vi "rango_dB.vi"(10 "rangosDB in":string[][](array[string])=[["50", "140"], ["40", "130"]], 11 "referencia[dB]":dbl format="%#_13g") -> (0 "tablaRef (Num)":dbl[](array[numeric]), 2 "Referencia[dB]":string[](array[string]), 3 "rango[dB]":string[](array[string]))   [LabVIEW 2019, in "Prueba07.lvclass"]
uses:
  Prueba07.lvclass
panel:
  out "ref_BD":string[](array[string])
  out "ref_NivMax":string[](array[string])
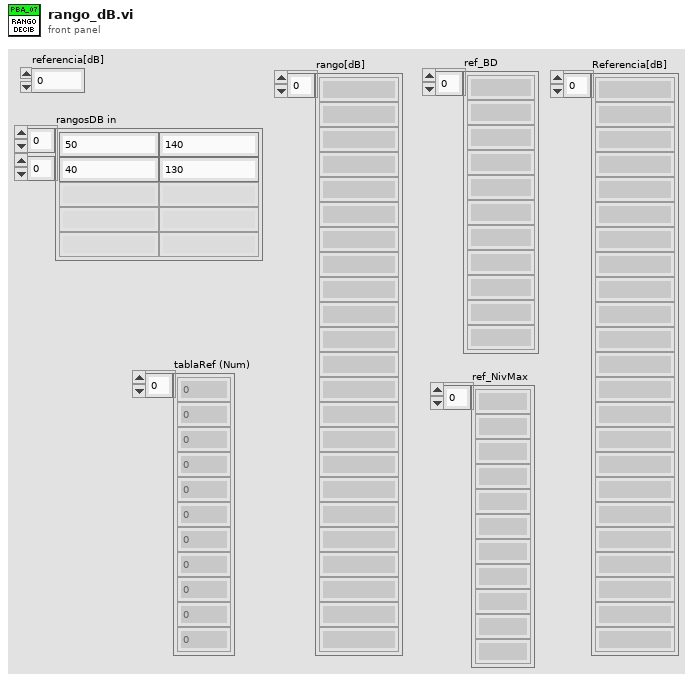
[diagram p1: front panel]
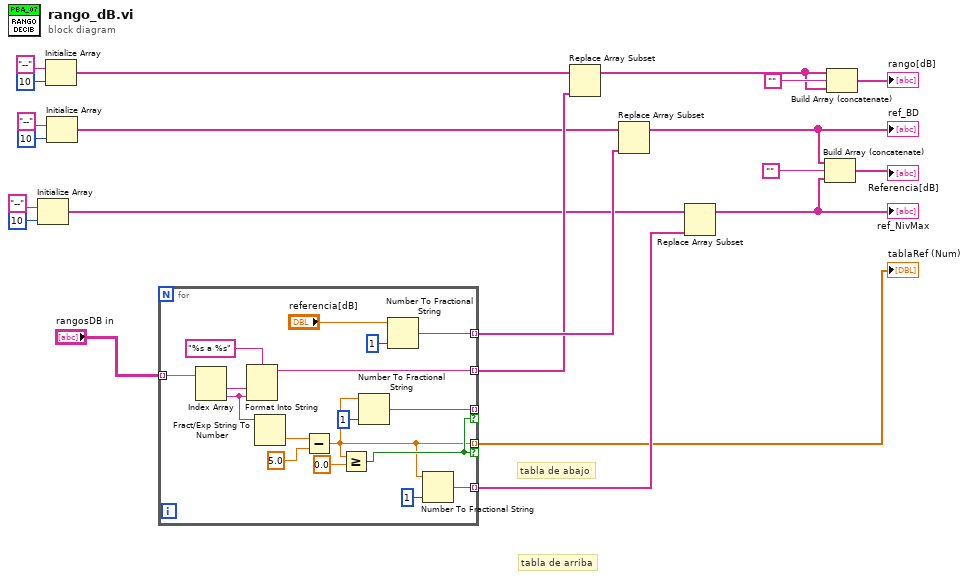
[diagram p0: block diagram]
diagram:
  # "tabla de abajo"
  # "tabla de arriba"
  n1 = Initialize Array("--" ("format string"), 10 ("dimension size")) -> (w6:string[])
  n2 = Initialize Array("--" ("format string"), 10 ("dimension size")) -> (w4:string[])
  n3 = Initialize Array("--" ("format string"), 10 ("dimension size")) -> (w5:string[])
  n4 = for {
    tunnel: "rangosDB in" -> [w38] mode=indexing
    tunnel: [w35] -> w12 mode=indexing
    tunnel: [w26] -> w17 mode=indexing if=w28
    tunnel: [w29] -> _ mode=indexing if=w28
    tunnel: [w25] -> w18 mode=indexing
    tunnel: [w22] -> w15 mode=indexing
    n5 = Index Array(array=w38) -> (element #1=w37:string, element #2=w34:string)  [unwired: 2 in]
    n6 = Format Into String(format string="%s a %s", w37, w34) -> (resulting string=w35:string)  [unwired: 2 in, 1 out]
    n7 = Fract/Exp String To Number(string=w34) -> (number=w33:dbl)  [unwired: 3 in, 1 out]
    n8 = Subtract(x=w33, y=5.0) -> (x-y=w26:dbl)
    n9 = Greater Or Equal?(x=w26, y=0.0) -> (x >= y?=w28:bool)
    n10 = Number To Fractional String(number=w26, precision (6)=i16 1) -> (F-format string=w29:string)  [unwired: 2 in]
    n11 = Number To Fractional String(number="referencia[dB]", precision (6)=i16 1) -> (F-format string=w22:string)  [unwired: 2 in]
    n12 = Number To Fractional String(number=w26, precision (6)=i16 1) -> (F-format string=w25:string)  [unwired: 2 in]
  }
  "tablaRef (Num)" <- w17
  n13 = Replace Array Subset(array=w4, new element=w12) -> (w2:string[])  [unwired: 1 in]
  n14 = Replace Array Subset(array=w5, new element=w15) -> (w11:string[])  [unwired: 1 in]
  "ref_BD" <- w11
  n15 = Replace Array Subset(array=w6, new element=w18) -> (w10:string[])  [unwired: 1 in]
  "ref_NivMax" <- w10
  n16 = Build Array (concatenate)(w11, "", w10) -> (→"Referencia[dB]":string[])
  n17 = Build Array (concatenate)(w2, "", w2) -> (→"rango[dB]":string[])
